vi "File.Load Subfolder to Zip File.vi"(8 "error in":errorcluster, 9 "Dest Path":path, 10 "Source Folder":path, 11 "Zip File":i64) -> (0 "error out":errorcluster, 2 "Dest Path Out":path, 3 "Zip File Out":i64)   [LabVIEW 2018]
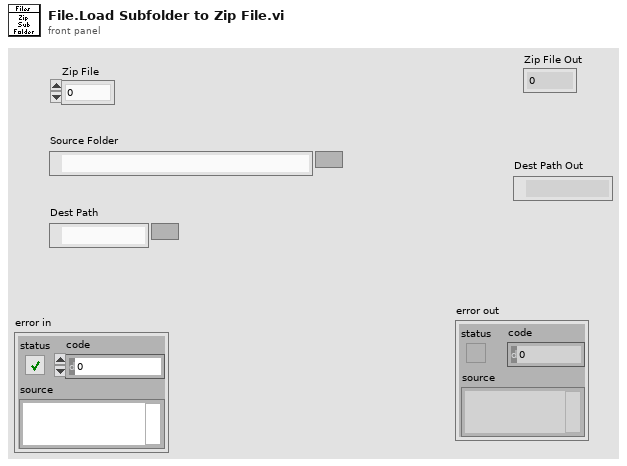
[diagram p1: front panel]
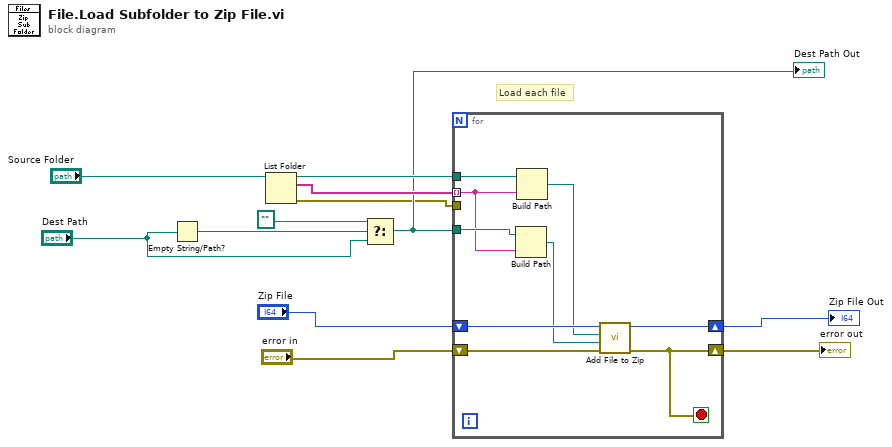
[diagram p0: block diagram]
diagram:
  # "Load each file"
  n1 = Empty String/Path?(string/path="Dest Path") -> (empty?=w5:bool)
  n2 = List Folder(path="Source Folder") -> (path out=w10:path, filenames=w11:string[], error out=w1:errorcluster)  [unwired: 3 in, 1 out]
  n3 = Select(t=path "" ("base path"), s=w5, f="Dest Path") -> (s? t:f=w2:path)
  "Dest Path Out" <- w2
  n4 = for {
    tunnel: w11 -> [w14] mode=indexing
    tunnel: w10 -> [w21]
    shift-right: [w13] -> w8
    shift-left: "error in" -> [w18]
    tunnel: w2 -> [w15]
    shift-right: [w16] -> w6
    shift-left: "Zip File" -> [w20]
    tunnel: w1 -> [_]
    stop <- w13 stop-if-true
    n5 = Build Path(base path=w15, name or relative path=w14) -> (appended path=w17:path)
    n6 = Build Path(base path=w21, name or relative path=w14) -> (appended path=w19:path)
    n7 = call <vilib>:"Add File to Zip.vi"("error in (no error)"=w18, "destination path in zip"=w17, "source file path"=w19, "zip file in"=w20) -> ("error out"=w13:errorcluster, "zip file out"=w16:i64)  [unwired: 6 in]
  }
  "error out" <- w8
  "Zip File Out" <- w6
